vi "FTW-Socket-Core-ValidateAddress.vi"(5 "Address":string, 7 "Allow wildcard replacement?":bool, 11 "error in":errorcluster) -> (6 "Sanitized Address":string, 8 "Message Transport Scheme":T1, 15 "error out":errorcluster)   [LabVIEW 2015]
uses:
  FTW-Socket-Core-TransportScheme.ctl
  regex/FTW-Regex-Execute.vi
  error/FTW-ERR-ThrowError.vi
  error/FTW-ERR-CallChain.vi
  error/FTW-ERR-NoErrorConstant.vi
  string/FTW-STR-ReplaceWhitespace.vi
  string/FTW-STR-Array-Delimit.vi
  regex/FTW-Regex-ReplaceAll.vi
  regex/FTW-Regex-Construct.vi
  lib/FTW-KernelFilepath.vi
  regex/FTW-Regex-Destroy.vi
panel:
  # "Inputs"
  # "Outputs"
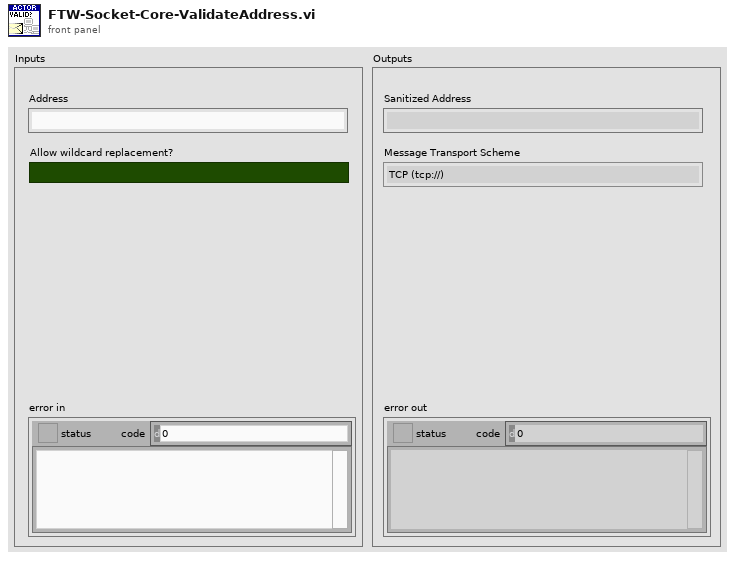
[diagram p1: front panel]
types:
  T1 = typedef "FTW-Socket-Core-TransportScheme.ctl" = enum16{"TCP (tcp://)", "Inter-Process (ipc://)", "In-Process (inproc://)", "WebSocket (ws://)"}
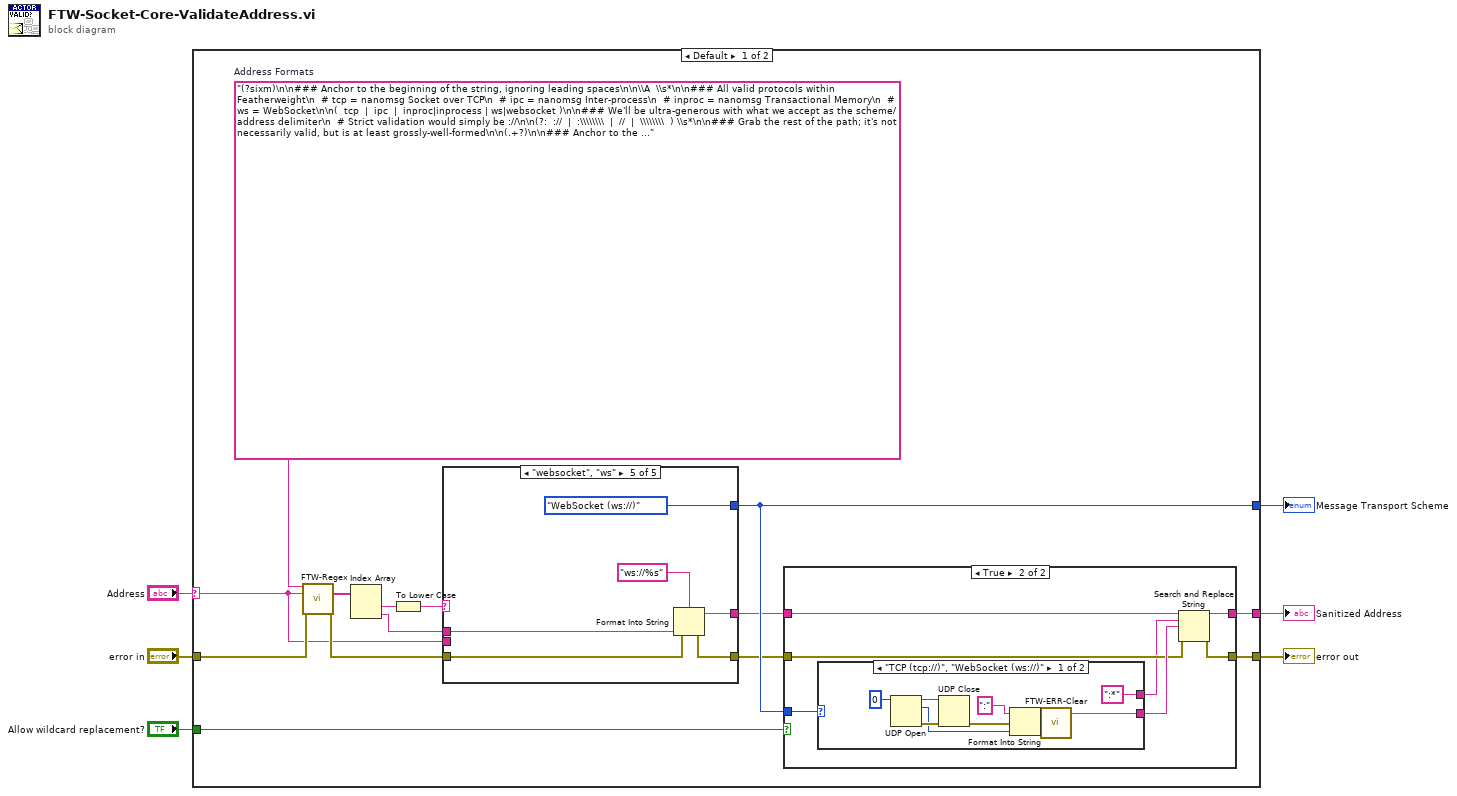
[diagram p0: block diagram]
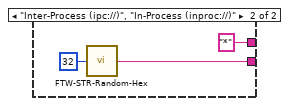
[diagram p3: hidden frame]
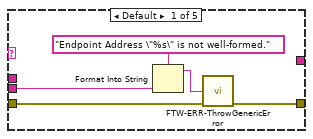
[diagram p4: hidden frame]
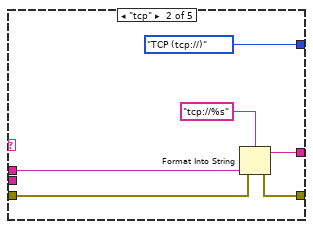
[diagram p5: hidden frame]
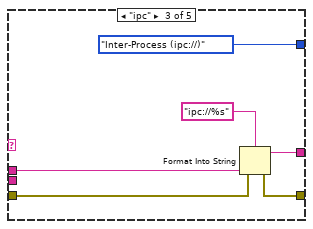
[diagram p6: hidden frame]
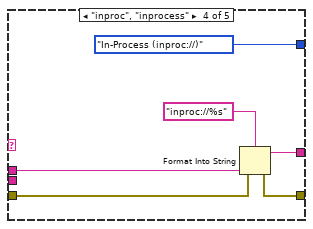
[diagram p7: hidden frame]
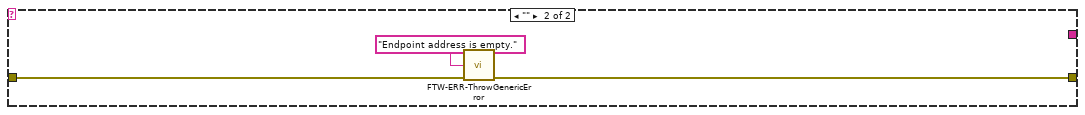
[diagram p8: hidden frame]
diagram:
  n1 = case shown="Default" "Address" {
    selector: "Address" -> [w13 _]
    tunnel: "error in" -> [w18 w73]
    tunnel: [w12 _] -> w5
    tunnel: [w8 _] -> w4
    tunnel: [w9 w72] -> w3
    tunnel: "Allow wildcard replacement?" -> [w7 _]
    frame Default {
      w20 = "(?sixm)\n\n### Anchor to the beginning of the string, ignoring leading spaces\n\n\\A  \\s*\n\n### All valid protocols within Featherweight\n  # tcp = nanomsg Socket over TCP\n  # ipc = nanomsg Inter-process\n  # inproc = nanomsg Transactional Memory\n  # ws = WebSocket\n\n(  tcp  |  ipc  |  inproc|inprocess | ws|websocket )\n\n### We'll be ultra-generous with what we accept as the scheme/address delimiter\n  # Strict validation would simply be ://\n\n(?:  ://  |  :\\\\\\\\  |  //  |  \\\\\\\\  ) \\s*\n\n### Grab the rest of the path; it's not necessarily valid, but is at least grossly-well-formed\n\n(.+?)\n\n### Anchor to the end of the string, ignoring trailing spaces\n\\s*\\z"  # Address Formats
      n2 = call "FTW-Regex.vi"("Regular Expression"=w20, "Input String"=w13, "error in"=w18) -> ("Submatches"=w19:string[], "error out"=w15:errorcluster)  [unwired: 8 in, 3 out]
      n3 = Index Array(array=w19) -> (element #1=w17:string, element #2=w14:string)  [unwired: 2 in]
      n4 = To Lower Case(string=w17) -> (all lower case string=w16:string)
      n5 = case shown="\"websocket\", \"ws\"" w16 {
        tunnel: [_ FTW-Socket-Core-TransportScheme."TCP (tcp://)" ("Message Transport Scheme") FTW-Socket-Core-TransportScheme."Inter-Process (ipc://)" ("Message Transport Scheme") FTW-Socket-Core-TransportScheme."In-Process (inproc://)" ("Message Transport Scheme") FTW-Socket-Core-TransportScheme."WebSocket (ws://)" ("Message Transport Scheme")] -> w12
        tunnel: w15 -> [w44 w47 w53 w59 w65]
        tunnel: w13 -> [w43 _ _ _ _]
        tunnel: [w42 w49 w55 w61 w67] -> w10
        tunnel: w14 -> [_ w48 w54 w60 w66]
        tunnel: [_ w50 w56 w62 w68] -> w11
        frame Default {
          n6 = Format Into String(format string="Endpoint Address \"%s\" is not well-formed." ("Error Message"), w43) -> (resulting string=w46:string)  [unwired: 2 in, 1 out]
          n7 = call "FTW-ERR-ThrowGenericError.vi"("Error Message"=w46, "error in"=w44) -> ("error out"=w42:errorcluster)  [unwired: 13 in]
        }
        frame "tcp" {
          n8 = Format Into String(format string="tcp://%s", error in=w47, w48) -> (resulting string=w50:string, error out=w49:errorcluster)  [unwired: 1 in]
        }
        frame "ipc" {
          n9 = Format Into String(format string="ipc://%s", error in=w53, w54) -> (resulting string=w56:string, error out=w55:errorcluster)  [unwired: 1 in]
        }
        frame "inproc", "inprocess" {
          n10 = Format Into String(format string="inproc://%s", error in=w59, w60) -> (resulting string=w62:string, error out=w61:errorcluster)  [unwired: 1 in]
        }
        frame "websocket", "ws" {
          n11 = Format Into String(format string="ws://%s", error in=w65, w66) -> (resulting string=w68:string, error out=w67:errorcluster)  [unwired: 1 in]
        }
      }
      n12 = case shown="True" w7 {
        tunnel: w12 -> [_ w29]
        tunnel: w11 -> [w22 w27]
        tunnel: w10 -> [w21 w26]
        tunnel: [w21 w25] -> w9
        tunnel: [w22 w24] -> w8
        frame False {
        }
        frame True {
          n13 = case shown="\"TCP (tcp://)\", \"WebSocket (ws://)\"" w29 {
            tunnel: [w32 w40] -> w28
            tunnel: [":*" "*"] -> w23
            frame "TCP (tcp://)", "WebSocket (ws://)" {
              n14 = UDP Open(11:u16 0 ("port")) -> (port=w37:refnum<k16>, 0:w36:errorcluster, 2:w34:u16)  [unwired: 4 in]
              n15 = UDP Close(connection ID=w37, 8:w36) -> (error out=w35:errorcluster)  [unwired: 1 out]
              n16 = Format Into String(initial string=":", error in=w35, w34) -> (resulting string=w32:string, error out=w33:errorcluster)  [unwired: 1 in]
              n17 = call "FTW-ERR-Clear.vi"("error to snuff"=w33) -> ()  [unwired: 1 out]
            }
            frame "Inter-Process (ipc://)", "In-Process (inproc://)" {
              n18 = call "FTW-STR-Random-Hex.vi"("String Length"=32) -> ("Random Hex String"=w40:string)  [unwired: 3 in]
            }
          }
          n19 = Search and Replace String(input string=w27, search string=w23, replace string=w28, error in=w26) -> (result string=w24:string, error out=w25:errorcluster)  [unwired: 4 in, 2 out]
        }
      }
    }
    frame "" {
      n20 = call "FTW-ERR-ThrowGenericError.vi"("Error Message"="Endpoint address is empty.", "error in"=w73) -> ("error out"=w72:errorcluster)  [unwired: 13 in]
    }
  }
  "error out" <- w3
  "Message Transport Scheme" <- w5
  "Sanitized Address" <- w4
